vi "BuildPackage.vi"(7 "ErrorCheck":enum16{"Csum", "CRC16"}(ring), 8 "error in":errorcluster caption="错误输入（无错误）", 9 "DataBytes":string, 10 "sequence":u8, 11 "TransferMode":T1) -> (0 "error out":errorcluster caption="错误输出", 3 "Packet":string)   [LabVIEW 2013]
uses:
  TransferMode.ctl
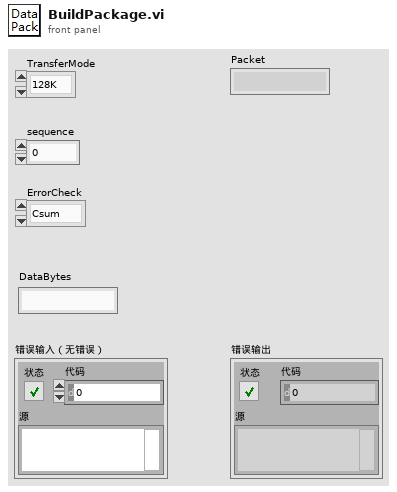
[diagram p1: front panel]
types:
  T1 = typedef "TransferMode.ctl" = enum16{"128K", "1024K"}
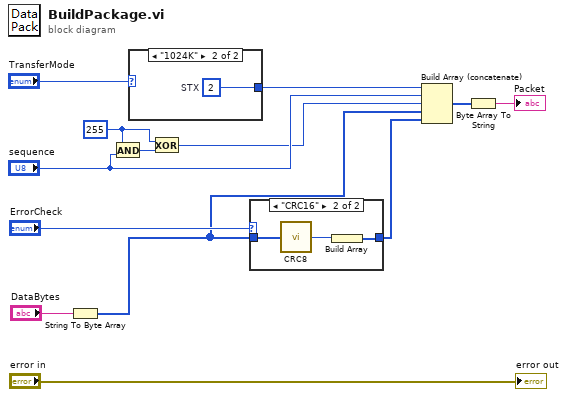
[diagram p0: block diagram]
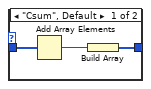
[diagram p2: hidden frame]
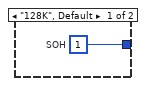
[diagram p3: hidden frame]
diagram:
  w9 = u8 255 ("STX")
  n1 = String To Byte Array(string="DataBytes") -> (unsigned byte array=w5:u8[])
  n2 = And(x=w9, y="sequence") -> (x .and. y?=w10:u8)
  n3 = case shown="\"1024K\"" "TransferMode" {
    tunnel: [w14 w15] -> w12
    frame "128K", Default {
      w14 = u8 1  # SOH
    }
    frame "1024K" {
      w15 = u8 2  # STX
    }
  }
  n4 = Exclusive Or(1:w10, 2:w9) -> (0:w8:u8)
  n5 = case shown="\"CRC16\"" "ErrorCheck" {
    tunnel: [w17 w19] -> w4
    tunnel: w5 -> [w16 w21]
    frame "Csum", Default {
      n6 = Add Array Elements(numeric array=w16) -> (sum=w18:u8)
      n7 = Build Array(w18) -> (w17:u8[])
    }
    frame "CRC16" {
      n8 = call "CRC8.vi"("DataByte"=w21) -> ("CRC"=w20:u8)
      n9 = Build Array(w20) -> (w19:u8[])
    }
  }
  n10 = Build Array (concatenate)(w12, "sequence", w8, w5, w4) -> (w3:u8[])
  n11 = Byte Array To String(unsigned byte array=w3) -> (string=→"Packet":string)
  "error out" <- "error in"
